vi "Connect-Disconnect.vi"(5 "Username":string, 6 "Password":string, 7 "Address":string, 8 "Error In":errorcluster) -> (0 "Error Out":errorcluster)   [LabVIEW 2018, in "Tests.lvlib" / "Agent.lvlib"]
uses:
  Agent.lvlib
  <vilib>/addons/_JKI Toolkits/Caraya/classes/Test/Test.lvclass
  <vilib>/addons/_JKI Toolkits/Caraya/classes/Assert/Assert.lvclass
  src/Toolkit/Agent/Agent.lvclass
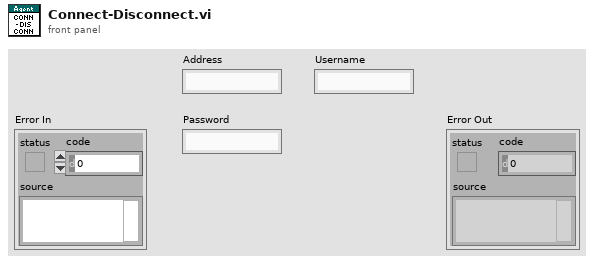
[diagram p1: front panel]
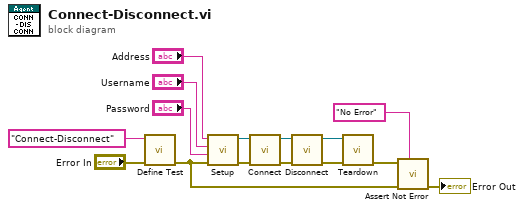
[diagram p0: block diagram]
diagram:
  n1 = call <vilib>:"Define Test.vi"("error in (no error)"="Error In", "Label (VI Title)"="Connect-Disconnect") -> ("error out"=w11:errorcluster)  [unwired: 9 in]
  n2 = call "Setup.vi"("Error In"=w11, "Password"="Password", "Username"="Username", "Address"="Address") -> ("Error Out"=w5:errorcluster, "Agent"=w6:refnum<class "Agent.lvclass">)  [unwired: 6 in]
  n3 = call "Connect.vi"("Error In"=w5, "Agent In"=w6) -> ("Error Out"=w3:errorcluster, "Agent Out"=w4:refnum<class "Agent.lvclass">)  [unwired: 8 in]
  n4 = call "Disconnect.vi"("Error In"=w3, "Agent In"=w4) -> ("Error Out"=w1:errorcluster, "Agent Out"=w2:refnum<class "Agent.lvclass">)  [unwired: 8 in]
  n5 = call "Teardown.vi"("Error In"=w1, "Agent"=w2) -> ("Error Out"=w10:errorcluster)  [unwired: 9 in]
  n6 = call <vilib>:"Assert Not Error.vi"("Label"="No Error", "error in (no error)"=w11, "Not Error?"=w10) -> ("error out"=→"Error Out":errorcluster)  [unwired: 8 in]
